vi "flow_event_add.vi"(0 "user_event in":refnum<user-event>, 11 "error in (no error)":errorcluster caption="エラー入力（エラーなし）") -> (4 "user_event out":refnum<user-event>, 15 "error out":errorcluster caption="エラー出力")   [LabVIEW 2015]
uses:
  flow_queue_datatype.ctl
  flow_event_datatype.ctl
panel:
  in  "data":T1
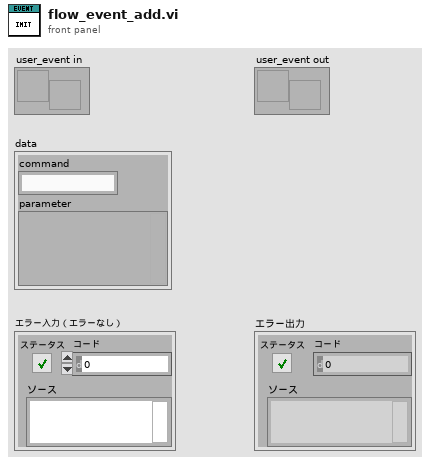
[diagram p1: front panel]
types:
  T1 = typedef "flow_event_datatype.ctl" = cluster{"command":string, "parameter":variant}
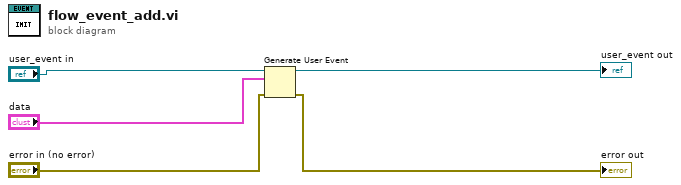
[diagram p0: block diagram]
diagram:
  n1 = Generate User Event(user event="user_event in", event data cluster="data", error in="error in (no error)") -> (user event out=→"user_event out":refnum<user-event>, error out=→"error out":errorcluster)  [unwired: 1 in]
